vi "Redirect Assemblies in TestStand Palette ini File.vi"() -> ()   [LabVIEW 2013, in "Assembly Redirection VIs.lvlib"]
uses:
  Assembly Redirection VIs.lvlib
  <vilib>/xml/Load XML File.vi
  <vilib>/xml/Close Reference(Node).vi
  <vilib>/xml/Close Reference(NNMap).vi
  <resource>/objmgr/DOMUserDefRef.rc
  <vilib>/xml/NI_XML.lvlib
  <vilib>/ni/Simple XML/Simple XML.lvlib
panel:
  in  "New VS InstallPath":string="C:\\Program Files (x86)\\National Instruments\\VeriStand 2013"
  in  "New Steps Version String":string="13.0.4.0"
  in  "New TS ini File Location":path=path "C:/Users/Public/Documents/Git-Source/VeriStand-Custom-Steps-For-TestStand/Source/TestStand Custom Steps ini Files/NI_VeristandTypes_mod.ini"
  in  "New VS Assembly Version":string="2016.0.0.0"
  out "error out":errorcluster
  in  "Old TS ini File Location":path=path "C:/Users/Public/Documents/Git-Source/VeriStand-Custom-Steps-For-TestStand/Source/TestStand Custom Steps ini Files/NI_VeristandTypes.ini" caption="Source TS ini File Location"
  # "Arguments\n1: Old TS ini File Location\n2: New TS ini File Location\n3: New VS Assembly Version\n4: New Steps Version String\n5: New VS InstallPath"
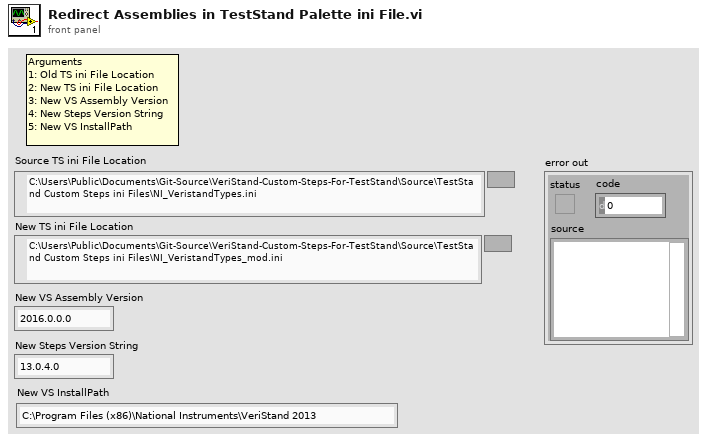
[diagram p1: front panel]
types:
  T1 = enum32{"invalid app kind", "Development System", "Run Time System", "Student Edition", "Embedded LabVIEW", "Evaluation", "Custom"}
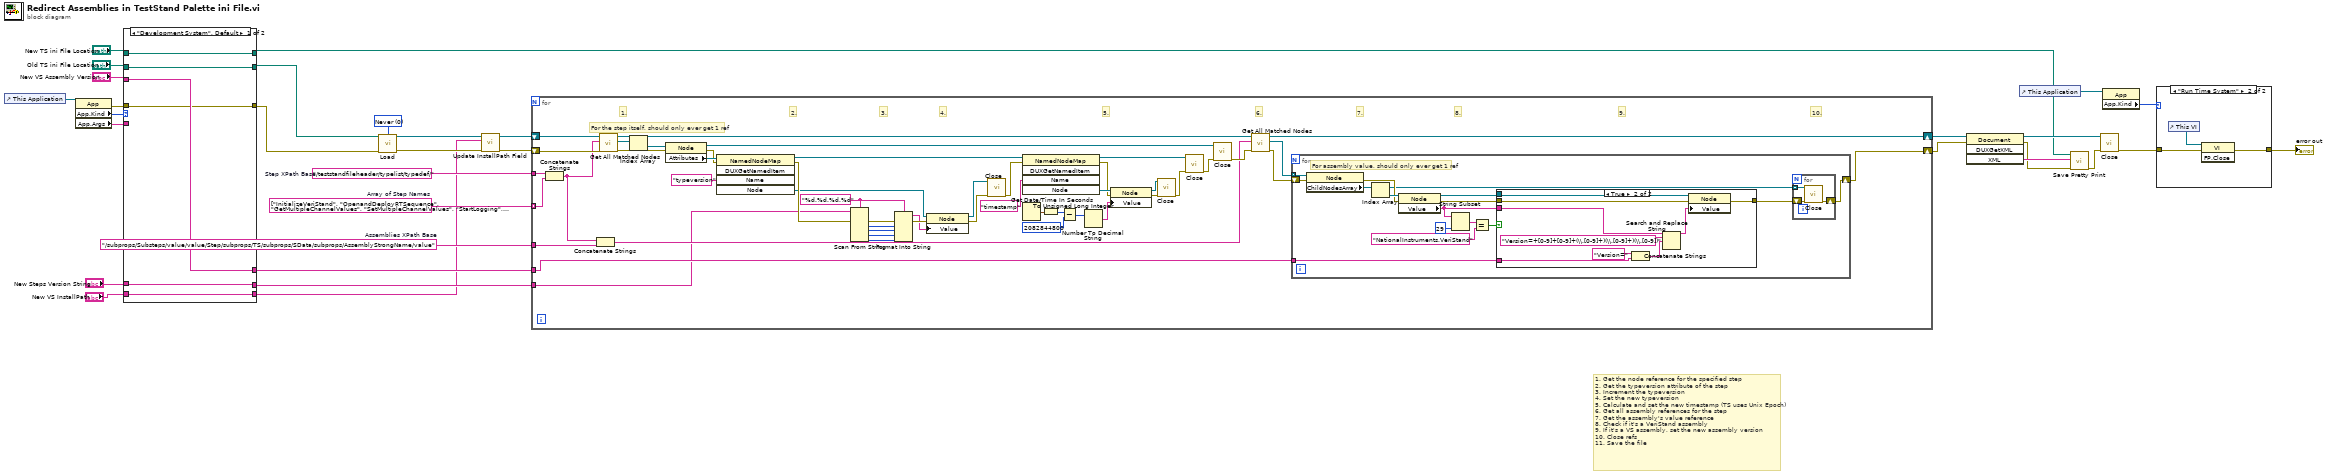
[diagram p0: block diagram]
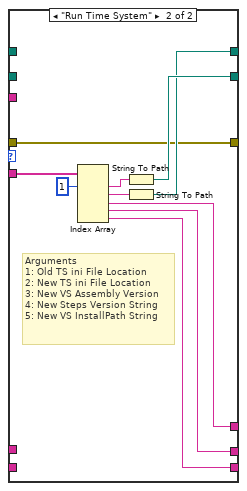
[diagram p3: hidden frame]
diagram:
  w3 = "/subprops/Substeps/value/value/Step/subprops/TS/subprops/SData/subprops/AssemblyStrongName/value"  # Assemblies XPath Base
  w26 = string[] ["InitializeVeriStand", "OpenandDeployRTSequence", "GetMultipleChannelValues", "SetMultipleChannelValues", "StartLogging", "StopLogging", "StopVeriStand", "RunProject", "ConnectProject", "DisconnectProject", "UndeployProject", "RunStimulusProfileAsynch", "DeployProject", "OpenReferences", "GetAlarmState", "SetChannelValue", "GetAlarmList", "RunStimulusProfileBlocking", "SetAlarmState", "SetModelParameterValue", "CloseProject", "UpdateModelParametersFromFile", "GetChannelValue", "LimitTestChannelValue", "GetChannelFaultValue", "GetModelParameterValue", "ClearFault", "ClearAllFaults", "PauseRTSequence", "StopRTSequence", "GetSequenceState", "GetAllSequenceNames", "StartRTSequence", "AbortRTSequence", "GetSequenceReturnValue", "StartStimulusProfileSession", "RunRTSequenceAction", "CloseWorkspace", "OpenWorkspace", "SilentConnect", "SilentDisconnect", "OpenProject", "RunRTSequencePassFail", "RunRTSequenceNumericLimit", "SetChannelFaultValue", "StopVeristandGateway", "StartVeristand"]  # Array of Step Names
  w32 = "/teststandfileheader/typelist/typedef/"  # Step XPath Base
  w33 = 0 items=["Never", "Always", "Auto"] ("validate on load (Auto)")
  # "1. Get the node reference for the specified step\n2. Get the typeversion attribute of the step\n3. Increment the typeversion\n4. Set the new typeversion\n5. Calculate and set the new timestamp (TS uses Unix Epoch)\n6. Get all assembly references for the step\n7. Get the assembly's value reference\n8. Check if it's a VeriStand assembly\n9. If it's a VS assembly, set the new assembly version\n10. Close refs\n11. Save the file"
  n1 = control-ref of="This Application"() -> (w22:refnum<vi>)
  n2 = property class="App"(reference=w22) -> (error out=w5:errorcluster, "App.Kind"=w21:T1, "App.Args"=w20:string[])  [unwired: 1 in, 1 out]
  n3 = case shown="\"Development System\", Default" w21 {
    tunnel: "New VS Assembly Version" -> [w37 _]
    tunnel: "New TS ini File Location" -> [w39 _]
    tunnel: "Old TS ini File Location" -> [w38 _]
    tunnel: w20 -> [_ w49]
    tunnel: [w39 w44] -> w17
    tunnel: [w38 w46] -> w19
    tunnel: [w37 w43] -> w18
    tunnel: [w36 w42] -> w11
    tunnel: "New Steps Version String" -> [w36 _]
    tunnel: w5 -> [w35 w41]
    tunnel: [w35 w41] -> w4
    tunnel: [w34 w40] -> w1
    tunnel: "New VS InstallPath" -> [w34 _]
    frame "Development System", Default {
    }
    frame "Run Time System" {
      # "Arguments\n1: Old TS ini File Location\n2: New TS ini File Location\n3: New VS Assembly Version\n4: New Steps Version String\n5: New VS InstallPath String"
      n4 = Index Array(array=w49, index #1=1 ("index")) -> (element #1=w47:string, element #2=w45:string, element #3=w43:string, element #4=w42:string, element #5=w40:string)  [unwired: 4 in]
      n5 = String To Path(string=w47) -> (path=w46:path)
      n6 = String To Path(string=w45) -> (path=w44:path)
    }
  }
  n7 = call-poly <vilib>:"Load.vi"("path to XML document"=w19, "validate on load (Auto)"=w33, "error in (no error)"=w4) -> ("DOM document out"=w9:refnum<k20>, "error out"=w10:errorcluster)  [unwired: 10 in, 1 out]
  n8 = call "Update InstallPath Field.vi"("error in (no error)"=w10, "New VS InstallPath"=w1, "DOM document in"=w9) -> ("error out"=w8:errorcluster, "DOM document out"=w7:refnum<k20>)  [unwired: 7 in]
  n9 = for {
    tunnel: w26 -> [w95] mode=indexing
    shift-right: [w93] -> w31
    shift-left: w7 -> [w98]
    tunnel: w32 -> [w96]
    shift-right: [w86] -> w6
    shift-left: w8 -> [w97]
    tunnel: w3 -> [w91]
    tunnel: w18 -> [w54]
    tunnel: w11 -> [w51]
    w75 = "%d.%d.%d.%d" ("format string")
    # "10."
    # "9."
    # "8."
    # "7."
    # "6."
    # "5."
    # "4."
    # "3."
    # "2."
    # "1."
    # "For the step itself, should only ever get 1 ref"
    n10 = Concatenate Strings(w96, w95) -> (w90:string)
    n11 = Concatenate Strings(w90, w91) -> (w89:string)
    n12 = call <vilib>:"Get All Matched Nodes.vi"("error in (no error)"=w97, "XPath expression"=w90, "node in"=w98) -> ("error out"=w81:errorcluster, "node result array"=w85:refnum<k20>[], "node out"=w94:refnum<k20>)  [unwired: 6 in]
    n13 = Index Array(array=w85) -> (element=w84:refnum<k20>)  [unwired: 1 in]
    n14 = property class="Node"(reference=w84, error in=w81) -> (reference out=w59:refnum<k20>, error out=w82:errorcluster, "Attributes"=w83:refnum<k20>)
    n15 = invoke class="NamedNodeMap" method="DUXGetNamedItem"(reference=w83, error in=w82, "Name"="typeversion") -> (reference out=w74:refnum<k20>, error out=w52:errorcluster, "Node"=w50:refnum<k20>)  [unwired: 2 in, 2 out]
    n16 = Scan From String(format string=w75, input string=w51, error in=w52) -> (error out=w79:errorcluster, output 1=w78:i32, output 2=w77:i32, output 3=w76:i32, output 4=w53:i32)  [unwired: 5 in, 2 out]
    n17 = Format Into String(format string=w75, error in=w79, w78, w77, w76, w53) -> (resulting string=w72:string, error out=w73:errorcluster)  [unwired: 1 in]
    n18 = property class="Node"(reference=w50, error in=w73, "Value"=w72) -> (reference out=w70:refnum<k20>, error out=w71:errorcluster)
    n19 = call-poly <vilib>:"Close.vi"("error in (no error)"=w71, "node"=w70) -> ("error out"=w69:errorcluster)  [unwired: 7 in]
    n20 = invoke class="NamedNodeMap" method="DUXGetNamedItem"(reference=w74, error in=w69, "Name"="timestamp") -> (reference out=w62:refnum<k20>, error out=w66:errorcluster, "Node"=w67:refnum<k20>)  [unwired: 2 in, 2 out]
    n21 = Get Date/Time In Seconds() -> (seconds since 1Jan1904=w58:timestamp)
    n22 = To Unsigned Long Integer(number=w58) -> (unsigned 32bit integer=w57:u32)
    n23 = Subtract(x=w57, y=u32 2082844800) -> (x-y=w55:u32)
    n24 = Number To Decimal String(number=w55) -> (decimal integer string=w65:string)  [unwired: 1 in]
    n25 = property class="Node"(reference=w67, error in=w66, "Value"=w65) -> (reference out=w63:refnum<k20>, error out=w64:errorcluster)
    n26 = call-poly <vilib>:"Close.vi"("error in (no error)"=w64, "node"=w63) -> ("error out"=w61:errorcluster)  [unwired: 7 in]
    n27 = call-poly <vilib>:"Close.vi"("error in (no error)"=w61, "named node map"=w62) -> ("error out"=w60:errorcluster)  [unwired: 7 in]
    n28 = call-poly <vilib>:"Close.vi"("error in (no error)"=w60, "node"=w59) -> ("error out"=w92:errorcluster)  [unwired: 7 in]
    n29 = call <vilib>:"Get All Matched Nodes.vi"("error in (no error)"=w92, "XPath expression"=w89, "node in"=w94) -> ("error out"=w87:errorcluster, "node result array"=w88:refnum<k20>[], "node out"=w93:refnum<k20>)  [unwired: 6 in]
    n30 = for {
      tunnel: w88 -> [w113] mode=indexing
      shift-right: [w108] -> w86
      shift-left: w87 -> [w112]
      tunnel: w54 -> [w99]
      # "For assembly value, should only ever get 1 ref"
      n31 = property class="Node"(reference=w113, error in=w112) -> (error out=w110:errorcluster, "ChildNodesArray"=w109:refnum<k20>[])  [unwired: 1 out]
      n32 = Index Array(array=w109) -> (element=w111:refnum<k20>)  [unwired: 1 in]
      n33 = property class="Node"(reference=w111, error in=w110) -> (reference out=w105:refnum<k20>, error out=w106:errorcluster, "Value"=w104:string)
      n34 = String Subset(string=w104, length (rest)=29 ("length (rest)")) -> (substring=w102:string)  [unwired: 1 in]
      n35 = Equal?(x=w102, y="NationalInstruments.VeriStand" ("Node Value 2")) -> (x = y?=w100:bool)
      n36 = case shown="True" w100 {
        tunnel: w104 -> [_ w123]
        tunnel: [w114 w119] -> w107
        tunnel: w106 -> [w114 w117]
        tunnel: w105 -> [_ w116]
        tunnel: w99 -> [_ w115]
        frame False {
        }
        frame True {
          n37 = Concatenate Strings("Version=" ("replace string (\"\")"), w115) -> (w120:string)
          n38 = Search and Replace String(input string=w123, search string="Version=+[0-9]+[0-9]+(\\.[0-9]+)(\\.[0-9]+)(\\.[0-9])", replace string=w120) -> (result string=w118:string)  [unwired: 5 in, 3 out]
          n39 = property class="Node"(reference=w116, error in=w117, "Value"=w118) -> (error out=w119:errorcluster)  [unwired: 1 out]
        }
      }
      n40 = for {
        tunnel: w109 -> [w126] mode=indexing
        shift-right: [w124] -> w108
        shift-left: w107 -> [w125]
        n41 = call-poly <vilib>:"Close.vi"("error in (no error)"=w125, "node"=w126) -> ("error out"=w124:errorcluster)  [unwired: 7 in]
      }
    }
  }
  n42 = invoke class="Document" method="DUXGetXML"(reference=w31, error in=w6) -> (reference out=w28:refnum<k20>, error out=w29:errorcluster, "XML"=w30:string)  [unwired: 2 in, 1 out]
  n43 = control-ref of="This Application"() -> (w16:refnum<vi>)
  n44 = call <vilib>:"Save Pretty Print.vi"("error in (no error)"=w29, "Pretty XML String"=w30, "XML file path"=w17) -> ("error out"=w27:errorcluster)  [unwired: 7 in, 1 out]
  n45 = call-poly <vilib>:"Close.vi"("error in (no error)"=w27, "node"=w28) -> ("error out"=w14:errorcluster)  [unwired: 7 in]
  n46 = property class="App"(reference=w16) -> ("App.Kind"=w15:T1)  [unwired: 1 in, 2 out]
  n47 = case shown="\"Run Time System\"" w15 {
    tunnel: w14 -> [w127 w129]
    tunnel: [w127 w128] -> w13
    frame "Development System", Default {
    }
    frame "Run Time System" {
      n48 = control-ref of="This VI"() -> (w130:refnum<vi>)
      n49 = invoke class="VI" method="FP.Close"(reference=w130, error in=w129) -> (error out=w128:errorcluster)  [unwired: 1 in, 2 out]
    }
  }
  "error out" <- w13
